vi "pmu_Phasor Scale.vi"(9 "phasors in":csg[](array[numeric]), 10 "phasor units":u32[](array[numeric]), 11 "format":u16) -> (2 "phasor out of range":bool, 3 "phasor byte array":u8[](array[numeric]))   [LabVIEW 2013, in "NI_EP_PMU.lvlib"]
uses:
  <vilib>/addons/Electrical Power/PMU/NI_EP_PMU.lvlib
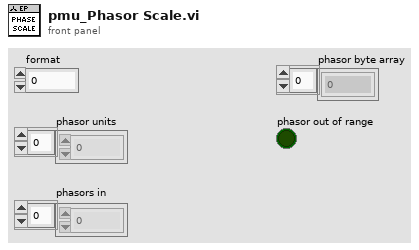
[diagram p1: front panel]
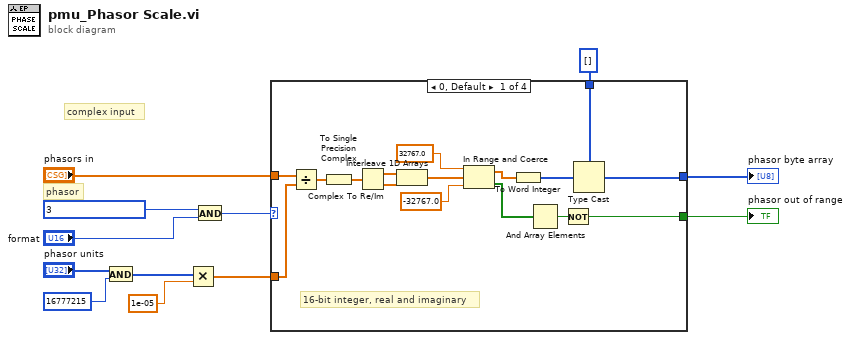
[diagram p0: block diagram]
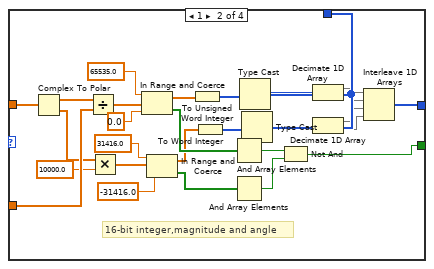
[diagram p2: hidden frame]
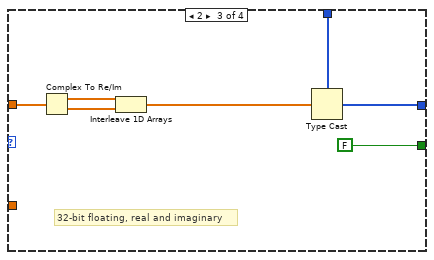
[diagram p3: hidden frame]
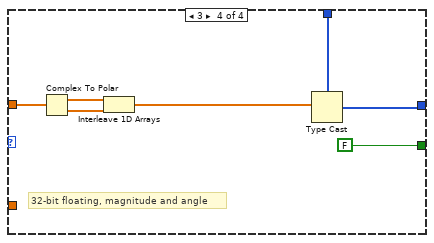
[diagram p4: hidden frame]
diagram:
  # "complex input"
  # "phasor"
  n1 = And(x="phasor units", y=u32 16777215) -> (x .and. y?=w4:u32[])
  n2 = Multiply(x=w4, y=1e-05) -> (x*y=w2:dbl[])
  n3 = And(x=u16 3, y="format") -> (x .and. y?=w10:u16)
  n4 = case shown="0, Default" w10 {
    tunnel: "phasors in" -> [w23 w56 w63 w70]
    tunnel: u8[] [] ("appended array") -> [w28 w37 w59 w66]
    tunnel: [w27 w30 w58 w65] -> w7
    tunnel: w2 -> [w22 w54 _ _]
    tunnel: [w13 w29 FALSE FALSE] -> w1
    frame 0, Default {
      # "16-bit integer, real and imaginary"
      n5 = Divide(x=w23, y=w22) -> (x/y=w21:cdb[])
      n6 = To Single Precision Complex(1:w21) -> (0:w20:csg[])
      n7 = Complex To Re/Im(x + iy=w20) -> (x=w26:sgl[], y=w25:sgl[])
      n8 = Interleave 1D Arrays(w26, w25) -> (w19:sgl[])
      n9 = In Range and Coerce(upper limit=sgl 32767.0, x=w19, lower limit=sgl -32767.0) -> (coerced(x)=w16:sgl[], In Range?=w15:bool[])
      n10 = To Word Integer(number=w16) -> (16bit integer=w24:i16[])
      n11 = And Array Elements(Boolean array=w15) -> (logical AND=w14:bool)
      n12 = Not(x=w14) -> (.not. x?=w13:bool)
      n13 = Type Cast(type=w28, x=w24) -> (*(type *) &x=w27:u8[])
    }
    frame 1 {
      # "16-bit integer,magnitude and angle"
      n14 = Complex To Polar(r * e^(i*theta)=w56) -> (r=w55:sgl[], theta=w53:sgl[])
      n15 = Divide(x=w55, y=w54) -> (x/y=w51:dbl[])
      n16 = Multiply(x=w53, y=sgl 10000.0) -> (x*y=w48:sgl[])
      n17 = In Range and Coerce(upper limit=65535.0, x=w51, lower limit=0.0) -> (coerced(x)=w42:dbl[], In Range?=w45:bool[])
      n18 = In Range and Coerce(upper limit=sgl 31416.0, x=w48, lower limit=sgl -31416.0) -> (coerced(x)=w41:sgl[], In Range?=w39:bool[])
      n19 = To Unsigned Word Integer(number=w42) -> (unsigned 16bit integer=w40:u16[])
      n20 = To Word Integer(number=w41) -> (16bit integer=w38:i16[])
      n21 = And Array Elements(Boolean array=w45) -> (logical AND=w44:bool)
      n22 = And Array Elements(Boolean array=w39) -> (logical AND=w43:bool)
      n23 = Type Cast(type=w37, x=w40) -> (*(type *) &x=w36:u8[])
      n24 = Type Cast(type=w37, x=w38) -> (*(type *) &x=w35:u8[])
      n25 = Not And(1:w43, 2:w44) -> (0:w29:bool)
      n26 = Decimate 1D Array(w36) -> (w34:u8[], w33:u8[])
      n27 = Decimate 1D Array(w35) -> (w32:u8[], w31:u8[])
      n28 = Interleave 1D Arrays(w34, w33, w32, w31) -> (w30:u8[])
    }
    frame 2 {
      # "32-bit floating, real and imaginary"
      n29 = Complex To Re/Im(x + iy=w63) -> (x=w62:sgl[], y=w61:sgl[])
      n30 = Interleave 1D Arrays(w62, w61) -> (w60:sgl[])
      n31 = Type Cast(type=w59, x=w60) -> (*(type *) &x=w58:u8[])
    }
    frame 3 {
      # "32-bit floating, magnitude and angle"
      n32 = Complex To Polar(r * e^(i*theta)=w70) -> (r=w69:sgl[], theta=w68:sgl[])
      n33 = Interleave 1D Arrays(w69, w68) -> (w67:sgl[])
      n34 = Type Cast(type=w66, x=w67) -> (*(type *) &x=w65:u8[])
    }
  }
  "phasor byte array" <- w7
  "phasor out of range" <- w1
